vi "Set Impedance Compensation.vi"(8 "error in (no error)":errorcluster, 10 "Impedance Compensation (0: None)":u32(ring) items=["None", "2 - Wire", "4 - Wire "], 11 "VISA resource name":refnum<visa-resource-name>) -> (0 "error out":errorcluster, 3 "VISA resource name out":refnum<visa-resource-name>)   [LabVIEW 2013, in "Fluke 5XXX Series Multicalibrators.lvlib"]
doc: "This VI activates or deactivates 2-wire or 4-wire impedance compensation. \n\nFour-wire and two-wire connections refer to methods of connecting the calibrator to the UUT to cancel out test lead resistance to assure the highest precision of the calibration output. The external sensing capability of the four-wire and two-wire compensated connections provide increased precision for resistance values below 110 kOhms and capacitance values 110 nF and above.\n\nNote:\n\nThe following 55xxA and 57xxA resistance modes are equivalent:\n\n55xxA 57xxA\nCOMP Off 2 wire Comp OFF, EX SNS off (disabled)\nCOMP 2 wire 2 wire Comp ON, EX SNS on (enabled)\nCOMP 4 wire 2 wire Comp OFF, EX SNS on (enabled)"
uses:
  Fluke 5XXX Series Multicalibrators.lvlib
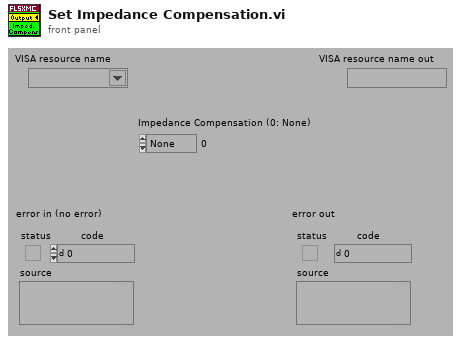
[diagram p1: front panel]
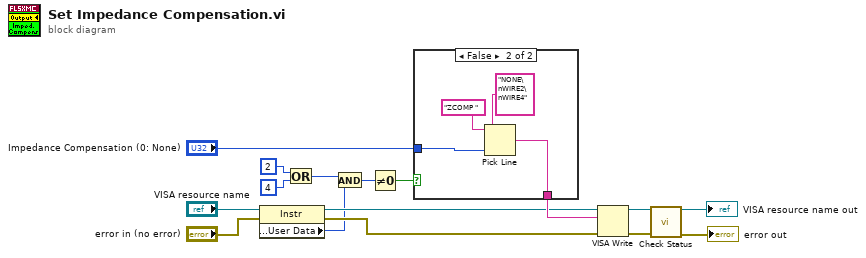
[diagram p0: block diagram]
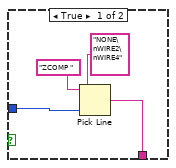
[diagram p2: hidden frame]
diagram:
  n1 = property class="Instr"(reference="VISA resource name", error in="error in (no error)") -> (reference out=w7:refnum<visa-resource-name>, error out=w5:errorcluster, "General Settings:User Data"=w4:u32)
  n2 = Or(x=u32 2 ("Numeric"), y=u32 4 ("Numeric")) -> (x .or. y?=w3:u32)
  n3 = And(x=w3, y=w4) -> (x .and. y?=w2:u32)
  n4 = Not Equal To 0?(x=w2) -> (x != 0?=w1:bool)
  n5 = case shown="False" w1 {
    tunnel: [w18 w22] -> w14
    tunnel: "Impedance Compensation (0: None)" -> [w17 w21]
    frame True {
      n6 = Pick Line(string ("")="ZCOMP ", multi-line string="NONE\nWIRE2\nWIRE4", line index=w17) -> (output string=w18:string)
    }
    frame False {
      n7 = Pick Line(string ("")="ZCOMP ", multi-line string="NONE\nWIRE2\nWIRE4", line index=w21) -> (output string=w22:string)
    }
  }
  n8 = VISA Write(VISA resource name=w7, write buffer=w14, error in (no error)=w5) -> (VISA resource name out=w16:refnum<visa-resource-name>, error out=w15:errorcluster)  [unwired: 1 out]
  n9 = call "Check Status.vi"("VISA resource name"=w16, "error in (no error)"=w15) -> ("VISA resource name out"=→"VISA resource name out":refnum<visa-resource-name>, "error out"=→"error out":errorcluster)  [unwired: 12 in]
